vi "DisplayTemp.vi"() -> ()   [LabVIEW 2017]
uses:
  <vilib>/Utility/file.llb/Write Delimited Spreadsheet (string).vi
panel:
  out "date/time string":string
  in  "file path (dialog if empty)":path
  out "Alarm":bool
  in  "Temp treshold":dbl
  out "Celsius Chart":cluster{"Temp treshold":dbl, "C temp":dbl}(graph)
  out "Celsius":dbl(slide) scale=0.0..100.0
  in  "C/F switch":bool
  out "Real\nactual time (ms)":u32
  out "Real \ncycle time (ms)":u32
  out "Computed\nactual time (ms)":u32
  in  "Max time (s)":dbl=10.0
  in  "stop":bool
  out "Farhenheit Chart":dbl(graph)
  out "Farhenheit":dbl(slide) scale=0.0..100.0
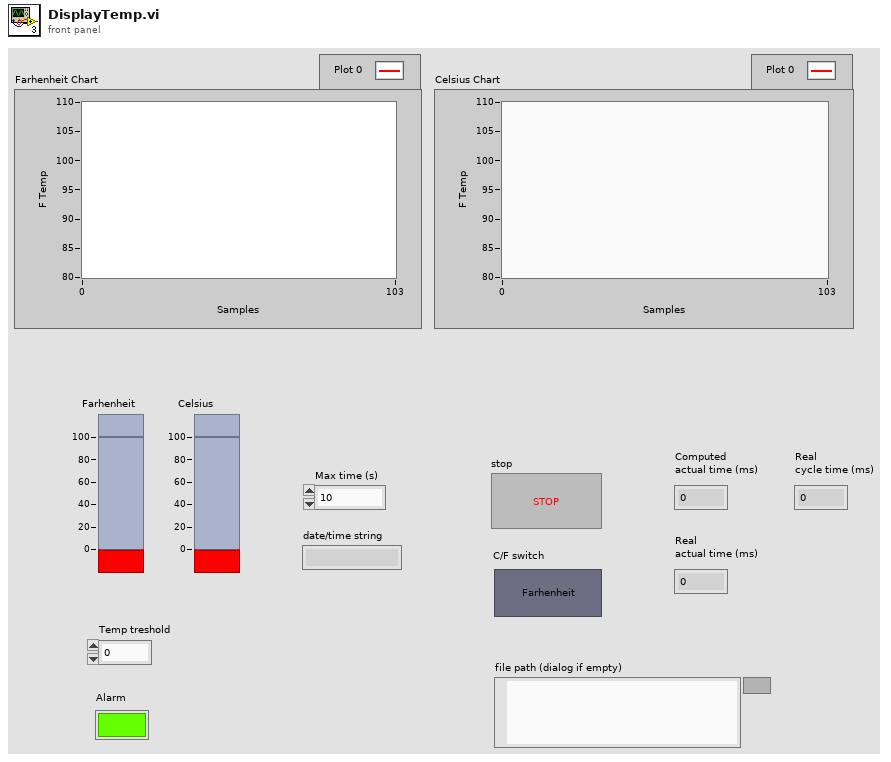
[diagram p1: front panel]
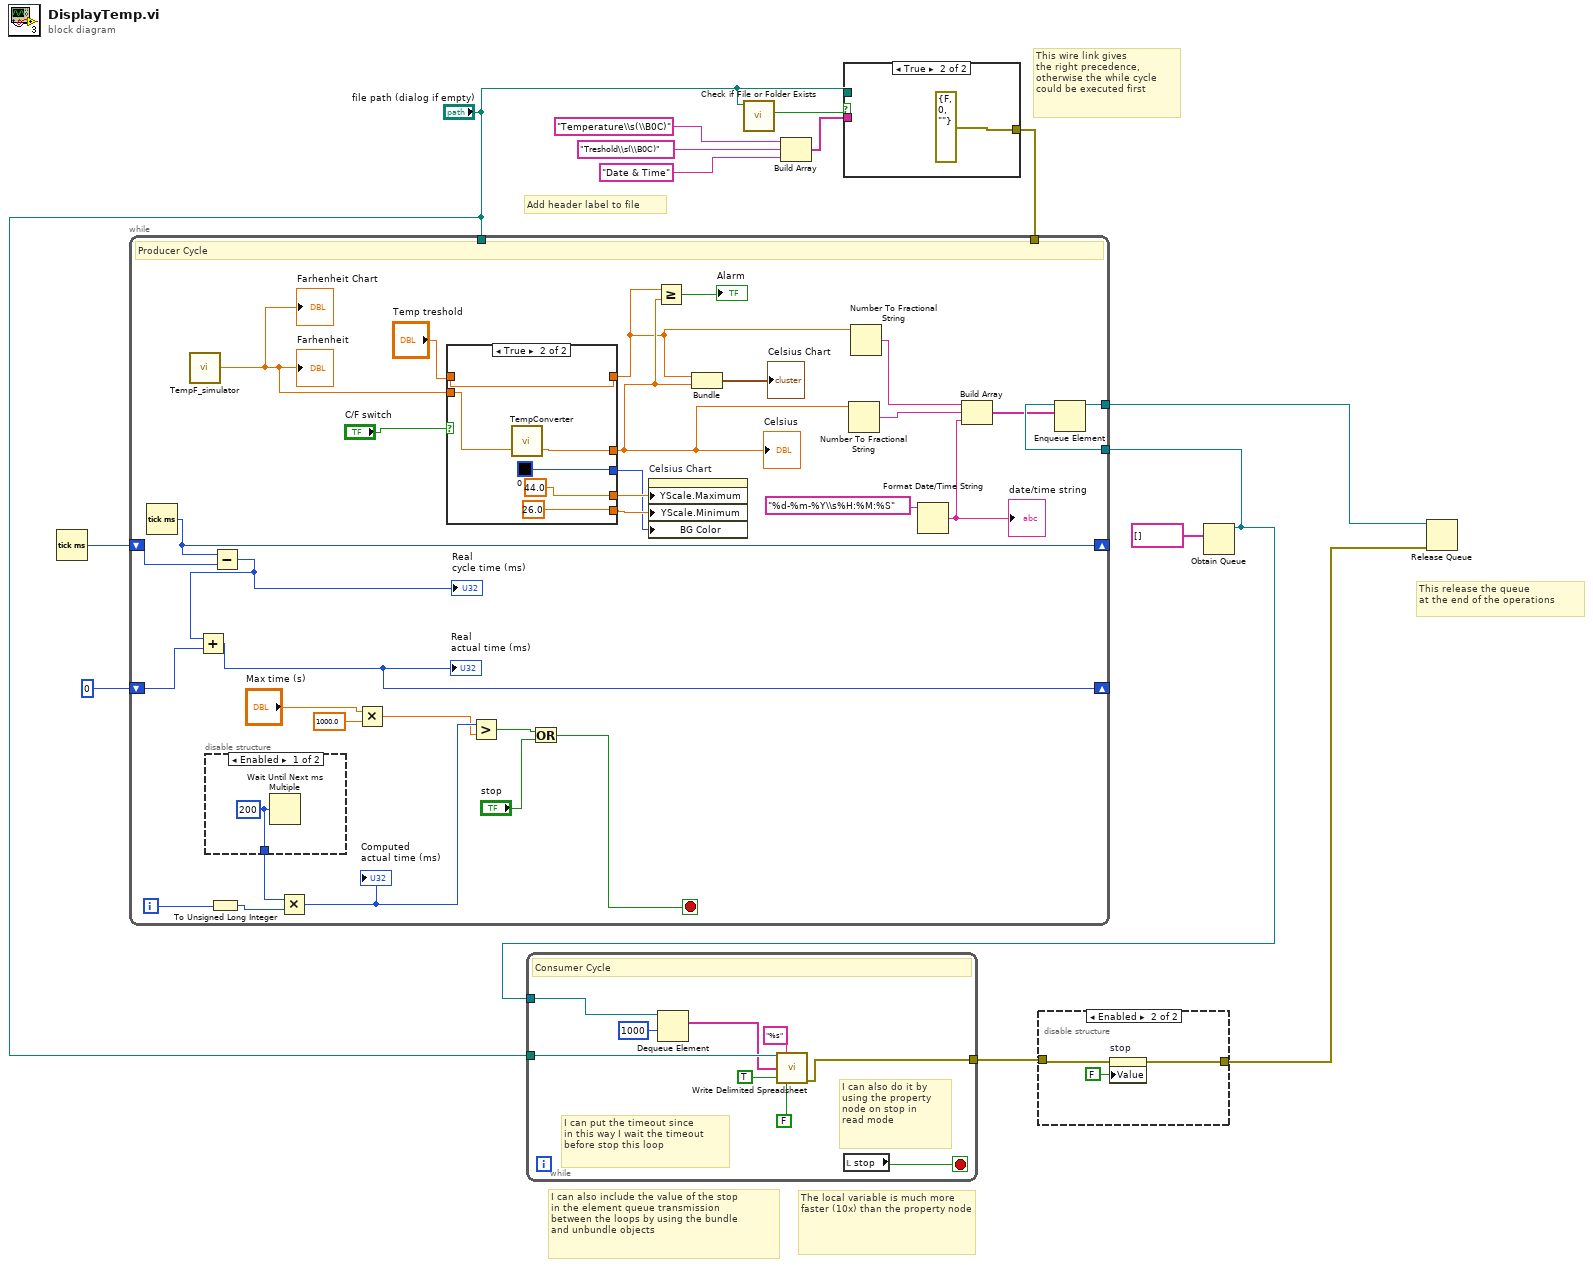
[diagram p0: block diagram]
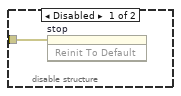
[diagram p2: hidden frame]
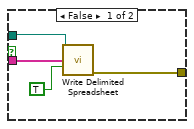
[diagram p3: hidden frame]
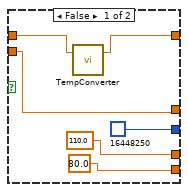
[diagram p4: hidden frame]
diagram:
  # "I can also include the value of the stop\nin the element queue transmission\nbetween the loops by using the bundle\nand unbundle objects"
  # "This release the queue\nat the end of the operations"
  # "The local variable is much more faster (10x) than the property node"
  # "This wire link gives\nthe right precedence,\notherwise the while cycle\ncould be executed first"
  # "Add header label to file"
  n1 = Tick Count (ms)() -> (millisecond timer value=w14:u32)
  n2 = call <vilib>:"Check if File or Folder Exists.vi"("path"="file path (dialog if empty)") -> ("file or folder exists?"=w7:bool)  [unwired: 8 in, 2 out]
  n3 = Build Array("Temperature\\s(\\B0C)", "Treshold\\s(\\B0C)" ("element"), "Date & Time" ("element")) -> (w11:string[])
  n4 = case shown="True" w7 {
    tunnel: w11 -> [w18 _]
    tunnel: "file path (dialog if empty)" -> [w17 _]
    tunnel: [w15 errorcluster {"status"=FALSE, "code"=0, "source"=""} ("error out")] -> w8
    frame False {
      n5 = call-poly <vilib>:"Write Delimited Spreadsheet.vi"("file path (dialog if empty)"=w17, "1D data"=w18, "append to file? (new file:F)"=TRUE) -> ("error out"=w15:errorcluster)  [unwired: 11 in, 1 out]
    }
    frame True {
    }
  }
  n6 = Obtain Queue(element data type=string[] []) -> (queue out=w4:refnum<queue>)  [unwired: 4 in, 2 out]
  n7 = while {
    shift-right: [w41] -> _
    shift-left: w14 -> [w42]
    shift-right: [w38] -> _
    shift-left: 0 -> [w40]
    tunnel: "file path (dialog if empty)" -> [_]
    tunnel: w8 -> [_]
    tunnel: w4 -> [w23]
    tunnel: [w20] -> w2
    i -> [w45]
    stop <- w21 stop-if-true
    # "Producer Cycle"
    n8 = Tick Count (ms)() -> (millisecond timer value=w41:u32)
    n9 = call "TempF_simulator.vi"() -> ("Farhenheit"=w36:dbl)  [unwired: 1 in]
    "Farhenheit" <- w36
    "Farhenheit Chart" <- w36
    n10 = disable-structure shown="Enabled" {
      disable-tunnel: [w64 _] -> w48
      frame Enabled {
        w64 = u32 200 ("millisecond multiple")
        n11 = Wait Until Next ms Multiple(millisecond multiple=w64) -> ()  [unwired: 1 out]
      }
      frame Disabled {
      }
    }
    n12 = To Unsigned Long Integer(number=w45) -> (unsigned 32bit integer=w44:u32)
    n13 = Subtract(x=w41, y=w42) -> (x-y=w39:u32)
    "Real \ncycle time (ms)" <- w39
    n14 = Add(x=w39, y=w40) -> (x+y=w38:u32)
    "Real\nactual time (ms)" <- w38
    n15 = Multiply(x=w48, y=w44) -> (x*y=w46:u32)
    "Computed\nactual time (ms)" <- w46
    n16 = Multiply(x="Max time (s)", y=1000.0) -> (x*y=w43:dbl)
    n17 = case shown="True" "C/F switch" {
      tunnel: w36 -> [w57 w63]
      tunnel: [w57 w62] -> w27
      tunnel: "Temp treshold" -> [w56 w61]
      tunnel: [w55 w61] -> w26
      tunnel: [110.0 44.0] -> w32
      tunnel: [80.0 26.0] -> w31
      tunnel: [u32 16448250 ("Color Box") u32 0 ("Color Box")] -> w30
      frame False {
        n18 = call "TempConverter.vi"("C temp"=w56) -> ("F temp"=w55:dbl)  [unwired: 1 in, 1 out]
      }
      frame True {
        n19 = call "TempConverter.vi"("F temp"=w63) -> ("C temp"=w62:dbl)  [unwired: 1 in, 1 out]
      }
    }
    "Celsius" <- w27
    n20 = Greater?(x=w46, y=w43) -> (0:w49:bool)
    n21 = Or(x=w49, y="stop") -> (x .or. y?=w21:bool)
    n22 = property on="Celsius Chart" class="WFChart (strict)"("YScale.Maximum"=w32, "YScale.Minimum"=w31, "BG Color"=w30) -> ()  [unwired: 2 in, 2 out]
    n23 = Greater Or Equal?(x=w26, y=w27) -> (x >= y?=→"Alarm":bool)
    n24 = Bundle("Temp treshold"=w26, "C temp"=w27) -> (→"Celsius Chart":cluster{"Temp treshold":dbl, "C temp":dbl})  [unwired: 1 in]
    n25 = Number To Fractional String(number=w27) -> (F-format string=w25:string)  [unwired: 3 in]
    n26 = Number To Fractional String(number=w26) -> (F-format string=w24:string)  [unwired: 3 in]
    n27 = Format Date/Time String(time format string (%c)="%d-%m-%Y\\s%H:%M:%S") -> (date/time string=w28:string)  [unwired: 2 in]
    "date/time string" <- w28
    n28 = Build Array(w24, w25, w28) -> (w22:string[])
    n29 = Enqueue Element(queue=w23, element=w22) -> (queue out=w20:refnum<queue>)  [unwired: 2 in, 2 out]
  }
  n30 = while {
    tunnel: "file path (dialog if empty)" -> [w70]
    tunnel: w4 -> [w69]
    tunnel: [w66] -> w3
    stop <- w65 stop-if-true
    # "I can also do it by\nusing the property\nnode on stop in \nread mode"
    # "I can put the timeout since\nin this way I wait the timeout\nbefore stop this loop"
    # "Consumer Cycle"
    n31 = Dequeue Element(queue=w69, timeout in ms (-1)=1000) -> (element=w68:string[])  [unwired: 1 in, 3 out]
    n32 = call-poly <vilib>:"Write Delimited Spreadsheet.vi"("file path (dialog if empty)"=w70, "format (%s)"="%s" ("format (%.3f)"), "1D data"=w68, "append to file? (new file:F)"=TRUE, "transpose? (no:F)"=FALSE) -> ("error out"=w66:errorcluster)  [unwired: 9 in, 1 out]
    n33 = local read "stop"() -> (w65:bool)
  }
  n34 = disable-structure shown="Enabled" {
    disable-tunnel: w3 -> [w74 w77]
    disable-tunnel: [_ w75] -> w1
    frame Disabled {
      n35 = invoke on="stop" class="Bool (strict)" method="Reinit To Default"(error in=w74) -> ()  [unwired: 2 in, 3 out]
    }
    frame Enabled {
      n36 = property on="stop" class="Bool (strict)"(error in=w77, "Value"=FALSE ("stop")) -> (error out=w75:errorcluster)  [unwired: 1 in, 1 out]
    }
  }
  n37 = Release Queue(queue=w2, error in (no error)=w1) -> ()  [unwired: 1 in, 3 out]
